vi "Array(DBL)ToFile_v2.vi"(0 "name_base":string="seqOUT", 1 "identifier(\"\")":string="trial01~000", 3 "extension (\".psv\")":string=".psv", 4 "1D-Array":dbl[](array[numeric])=[25.0, 55.0, 73.0, 90.0, 25.0, 55.0, 73.0, 90.0, 25.0, 55.0, 73.0, 90.0, 25.0, 55.0, 73.0, 90.0, 25.0, 55.0, 73.0, 90.0, 25.0, 55.0, 73.0, 90.0, 25.0, 55.0, 73.0, 90.0, 25.0, 55.0, 73.0, 90.0, 25.0, 55.0, 73.0, 90.0, 25.0, 55.0, 73.0, 90.0, 25.0, 55.0, 73.0, 90.0, 25.0, 55.0, 73.0, 90.0, 25.0, 55.0, 73.0, 90.0, 25.0, 55.0, 73.0, 90.0, 25.0, 55.0, 73.0, 90.0, 25.0, 55.0, 73.0, 90.0, 25.0, 55.0, 73.0, 90.0, 25.0, 55.0, 73.0, 90.0, 25.0, 55.0, 73.0, 90.0, 25.0, 55.0, 73.0, 90.0, 25.0, 55.0, 73.0, 90.0, 25.0, 55.0, 73.0, 90.0, 25.0, 55.0, 73.0, 90.0, 25.0, 55.0, 73.0, 90.0, 25.0, 55.0, 73.0, 90.0, 25.0, 55.0, 73.0, 90.0, 25.0, 55.0, 73.0, 90.0, 25.0, 55.0, 73.0, 90.0, 25.0, 55.0, 73.0, 90.0, 25.0, 55.0, 73.0, 90.0, 25.0, 55.0, 73.0, 90.0, 25.0, 55.0, 73.0, 90.0, 25.0, 55.0, 73.0, 90.0, 25.0, 55.0, 73.0, 90.0, 25.0, 55.0, 73.0, 90.0, 25.0, 55.0, 73.0, 90.0, 25.0, 55.0, 73.0, 90.0, 25.0, 55.0, 73.0, 90.0, 25.0, 55.0, 73.0, 90.0, 25.0, 55.0, 73.0, 90.0, 25.0, 55.0, 73.0, 90.0, 25.0, 55.0, 73.0, 90.0, 25.0, 55.0, 73.0, 90.0, 25.0, 55.0, 73.0, 90.0, 25.0, 55.0, 73.0, 90.0, 25.0, 55.0, 73.0, 90.0, 25.0, 55.0, 73.0, 90.0, 25.0, 55.0, 73.0, 90.0, 25.0, 55.0, 73.0, 90.0, 25.0, 55.0, 73.0, 90.0, 25.0, 55.0, 73.0, 90.0, 25.0, 55.0, 73.0, 90.0, 25.0, 55.0, 73.0, 90.0, 25.0, 55.0, 73.0, 90.0, 25.0, 55.0, 73.0, 90.0, 25.0, 55.0, 73.0, 90.0, 25.0, 55.0, 73.0, 90.0, 25.0, 55.0, 73.0, 90.0, 25.0, 55.0, 73.0, 90.0, 25.0, 55.0, 73.0, 90.0, 25.0, 55.0, 73.0, 90.0, 25.0, 55.0, 73.0, 90.0, 25.0, 55.0, 73.0, 90.0, 25.0, 55.0, 73.0, 90.0, 25.0, 55.0, 73.0, 90.0, 25.0, 55.0, 73.0, 90.0, 25.0, 55.0, 73.0, 90.0, 25.0, 55.0, 73.0, 90.0, 25.0, 55.0, 73.0, 90.0, 25.0, 55.0, 73.0, 90.0, 25.0, 55.0, 73.0, 90.0, 25.0, 55.0, 73.0, 90.0, 25.0, 55.0, 73.0, 90.0, 25.0, 55.0, 73.0, 90.0, 25.0, 55.0, 73.0, 90.0, 25.0, 55.0, 73.0, 90.0, 25.0, 55.0, 73.0, 90.0, 25.0, 55.0, 73.0, 90.0, 25.0, 55.0, 73.0, 90.0, 25.0, 55.0, 73.0, 90.0, 25.0, 55.0, 73.0, 90.0, 25.0, 55.0, 73.0, 90.0, 25.0, 55.0, 73.0, 90.0, 25.0, 55.0, 73.0, 90.0, 25.0, 55.0, 73.0, 90.0, 25.0, 55.0, 73.0, 90.0, 25.0, 55.0, 73.0, 90.0, 25.0, 55.0, 73.0, 90.0, 25.0, 55.0, 73.0, 90.0, 25.0, 55.0, 73.0, 90.0, 25.0, 55.0, 73.0, 90.0, 25.0, 55.0, 73.0, 90.0, 25.0, 55.0, 73.0, 90.0, 25.0, 55.0, 73.0, 90.0, 25.0, 55.0, 73.0, 90.0, 25.0, 55.0, 73.0, 90.0, 25.0, 55.0, 73.0, 90.0, 25.0, 55.0, 73.0, 90.0, 25.0, 55.0, 73.0, 90.0, 25.0, 55.0, 73.0, 90.0, 25.0, 55.0, 73.0, 90.0, 25.0, 55.0, 73.0, 90.0, 25.0, 55.0, 73.0, 90.0, 25.0, 55.0, 73.0, 90.0, 25.0, 55.0, 73.0, 90.0, 25.0, 55.0, 73.0, 90.0, 25.0, 55.0, 73.0, 90.0, 25.0, 55.0, 73.0, 90.0, 25.0, 55.0, 73.0, 90.0, 25.0, 55.0, 73.0, 90.0, 25.0, 55.0, 73.0, 90.0, 25.0, 55.0, 73.0, 90.0, 25.0, 55.0, 73.0, 90.0, 25.0, 55.0, 73.0, 90.0, 25.0, 55.0, 73.0, 90.0, 25.0, 55.0, 73.0, 90.0, 25.0, 55.0, 73.0, 90.0, 25.0, 55.0, 73.0, 90.0, 25.0, 55.0, 73.0, 90.0, 25.0, 55.0, 73.0, 90.0, 25.0, 55.0, 73.0, 90.0, 25.0, 55.0, 73.0, 90.0, 25.0, 55.0, 73.0, 90.0, 25.0, 55.0, 73.0, 90.0, 25.0, 55.0, 73.0, 90.0, 25.0, 55.0, 73.0, 90.0, 25.0, 55.0, 73.0, 90.0, 25.0, 55.0, 73.0, 90.0, 25.0, 55.0, 73.0, 90.0, 25.0, 55.0, 73.0, 90.0, 25.0, 55.0, 73.0, 90.0, 25.0, 55.0, 73.0, 90.0, 25.0, 55.0, 73.0, 90.0, 25.0, 55.0, 73.0, 90.0, 25.0, 55.0, 73.0, 90.0, 25.0, 55.0, 73.0, 90.0, 25.0, 55.0, 73.0, 90.0, 25.0, 55.0, 73.0, 90.0, 25.0, 55.0, 73.0, 90.0, 25.0, 55.0, 73.0, 90.0, 25.0, 55.0, 73.0, 90.0, 25.0, 55.0, 73.0, 90.0, 25.0, 55.0, 73.0, 90.0, 25.0, 55.0, 73.0, 90.0, 25.0, 55.0, 73.0, 90.0, 25.0, 55.0, 73.0, 90.0, 25.0, 55.0, 73.0, 90.0, 25.0, 55.0, 73.0, 90.0, 25.0, 55.0, 73.0, 90.0, 25.0, 55.0, 73.0, 90.0, 25.0, 55.0, 73.0, 90.0, 25.0, 55.0, 73.0, 90.0, 25.0, 55.0, 73.0, 90.0, 25.0, 55.0, 73.0, 90.0, 25.0, 55.0, 73.0, 90.0, 25.0, 55.0, 73.0, 90.0, 25.0, 55.0, 73.0, 90.0, 25.0, 55.0, 73.0, 90.0, 25.0, 55.0, 73.0, 90.0, 25.0, 55.0, 73.0, 90.0, 25.0, 55.0, 73.0, 90.0, 25.0, 55.0, 73.0, 90.0, 25.0, 55.0, 73.0, 90.0, 25.0, 55.0, 73.0, 90.0, 25.0, 55.0, 73.0, 90.0, 25.0, 55.0, 73.0, 90.0, 25.0, 55.0, 73.0, 90.0, 25.0, 55.0, 73.0, 90.0, 25.0, 55.0, 73.0, 90.0, 25.0, 55.0, 73.0, 90.0, 25.0, 55.0, 73.0, 90.0, 25.0, 55.0, 73.0, 90.0, 25.0, 55.0, 73.0, 90.0, 25.0, 55.0, 73.0, 90.0, 25.0, 55.0, 73.0, 90.0, 25.0, 55.0, 73.0, 90.0, 25.0, 55.0, 73.0, 90.0, 25.0, 55.0, 73.0, 90.0, 25.0, 55.0, 73.0, 90.0, 25.0, 55.0, 73.0, 90.0, 25.0, 55.0, 73.0, 90.0, 25.0, 55.0, 73.0, 90.0, 25.0, 55.0, 73.0, 90.0, 25.0, 55.0, 73.0, 90.0, 25.0, 55.0, 73.0, 90.0, 25.0, 55.0, 73.0, 90.0, 25.0, 55.0, 73.0, 90.0, 25.0, 55.0, 73.0, 90.0, 25.0, 55.0, 73.0, 90.0, 25.0, 55.0, 73.0, 90.0, 25.0, 55.0, 73.0, 90.0, 25.0, 55.0, 73.0, 90.0, 25.0, 55.0, 73.0, 90.0, 25.0, 55.0, 73.0, 90.0, 25.0, 55.0, 73.0, 90.0, 25.0, 55.0, 73.0, 90.0, 25.0, 55.0, 73.0, 90.0, 25.0, 55.0, 73.0, 90.0, 25.0, 55.0, 73.0, 90.0, 25.0, 55.0, 73.0, 90.0, 25.0, 55.0, 73.0, 90.0, 25.0, 55.0, 73.0, 90.0, 25.0, 55.0, 73.0, 90.0, 25.0, 55.0, 73.0, 90.0, 25.0, 55.0, 73.0, 90.0, 25.0, 55.0, 73.0, 90.0, 25.0, 55.0, 73.0, 90.0, 25.0, 55.0, 73.0, 90.0, 25.0, 55.0, 73.0, 90.0, 25.0, 55.0, 73.0, 90.0, 25.0, 55.0, 73.0, 90.0, 25.0, 55.0, 73.0, 90.0, 25.0, 55.0, 73.0, 90.0, 25.0, 55.0, 73.0, 90.0, 25.0, 55.0, 73.0, 90.0, 25.0, 55.0, 73.0, 90.0, 25.0, 55.0, 73.0, 90.0, 25.0, 55.0, 73.0, 90.0, 25.0, 55.0, 73.0, 90.0, 25.0, 55.0, 73.0, 90.0, 25.0, 55.0, 73.0, 90.0, 25.0, 55.0, 73.0, 90.0, 25.0, 55.0, 73.0, 90.0, 25.0, 55.0, 73.0, 90.0, 25.0, 55.0, 73.0, 90.0, 25.0, 55.0, 73.0, 90.0, 25.0, 55.0, 73.0, 90.0, 25.0, 55.0, 73.0, 90.0, 25.0, 55.0, 73.0, 90.0, 25.0, 55.0, 73.0, 90.0, 25.0, 55.0, 73.0, 90.0, 25.0, 55.0, 73.0, 90.0, 25.0, 55.0, 73.0, 90.0, 25.0, 55.0, 73.0, 90.0, 25.0, 55.0, 73.0, 90.0, 25.0, 55.0, 73.0, 90.0, 25.0, 55.0, 73.0, 90.0, 25.0, 55.0, 73.0, 90.0, 25.0, 55.0, 73.0, 90.0, 25.0, 55.0, 73.0, 90.0, 25.0, 55.0, 73.0, 90.0, 25.0, 55.0, 73.0, 90.0, 25.0, 55.0, 73.0, 90.0, 25.0, 55.0, 73.0, 90.0, 25.0, 55.0, 73.0, 90.0, 25.0, 55.0, 73.0, 90.0, 25.0, 55.0, 73.0, 90.0, 25.0, 55.0, 73.0, 90.0, 25.0, 55.0, 73.0, 90.0, 25.0, 55.0, 73.0, 90.0] format="%_8f", 5 "2D-Array":dbl[][](array[numeric])=array100x100[10000 elements] format="%_8f", 7 "Array Type (2D)":enum16{"2D", "row", "column"}(ring), 8 "Child Directory":path=path "SEQUENCES/OUT", 9 "delimiter (\"|\")":string="|", 11 "data format (DBL)":string="%.8f", 12 "Parent Directory":path=path "C:/misc/LabVIEW/FILES", 13 "Filename Collision Handling":T1(ring)) -> (20 "target_filepath":path=path "C:/misc/LabVIEW/FILES/SEQUENCES/OUT/seqOUT_trial01.psv", 23 "Saved":bool=TRUE, 25 "data_string":string="25\r\n55\r\n73\r\n90\r\n25\r\n55\r\n73\r\n90\r\n25\r\n55\r\n73\r\n90\r\n25\r\n55\r\n73\r\n90\r\n25\r\n55\r\n73\r\n90\r\n25\r\n55\r\n73\r\n90\r\n25\r\n55\r\n73\r\n90\r\n25\r\n55\r\n73\r\n90\r\n25\r\n55\r\n73\r\n90\r\n25\r\n55\r\n73\r\n90\r\n25\r\n55\r\n73\r\n90\r\n25\r\n55\r\n73\r\n90\r\n25\r\n55\r\n73\r\n90\r\n25\r\n55\r\n73\r\n90\r\n25\r\n55\r\n73\r\n90\r\n25\r\n55\r\n73\r\n90\r\n25\r\n55\r\n73\r\n90\r\n25\r\n55\r\n73\r\n90\r\n25\r\n55\r\n73\r\n90\r\n25\r\n55\r\n73\r\n90\r\n25\r\n55\r\n73\r\n90\r\n25\r\n55\r\n73\r\n90\r\n25\r\n55\r\n73\r\n90\r\n25\r\n55\r\n73\r\n90\r\n25\r\n55\r\n73\r\n90\r\n25\r\n55\r\n73\r\n90\r\n25\r\n55\r\n73\r\n90\r\n25\r\n55\r\n73\r\n90\r\n25\r\n55\r\n73\r\n90\r\n25\r\n55\r\n73\r\n90\r\n25\r\n55\r\n73\r\n90\r\n25\r\n55\r\n73\r\n90\r\n25\r\n55\r\n73\r\n90\r\n25\r\n55\r\n73\r\n90\r\n25\r\n55\r\n73\r\n90\r\n25\r\n55\r\n73\r\n90\r\n25\r\n55\r\n73\r\n90\r\n25\r\n55\r\n...")   [LabVIEW 2014]
panel:
  in  "?":enum32{"MAIN", "DATA"}(tab)
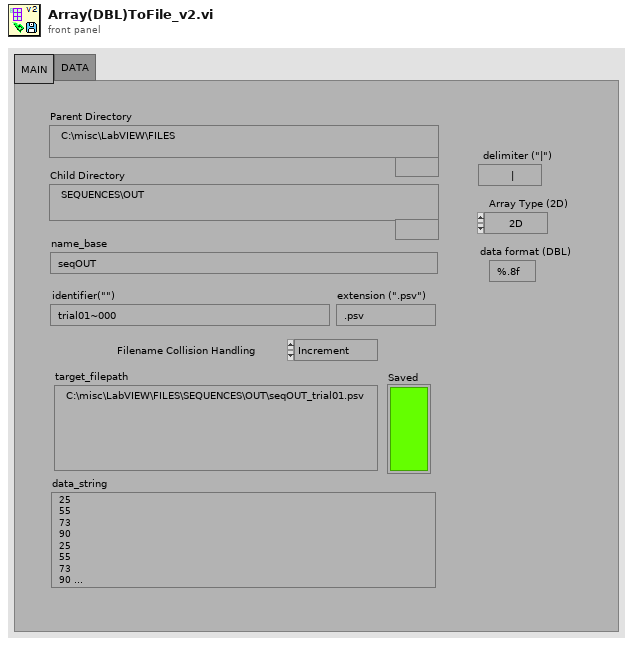
[diagram p1: front panel]
types:
  T1 = enum16{"Increment", "Overwrite", "Treat as Error"}
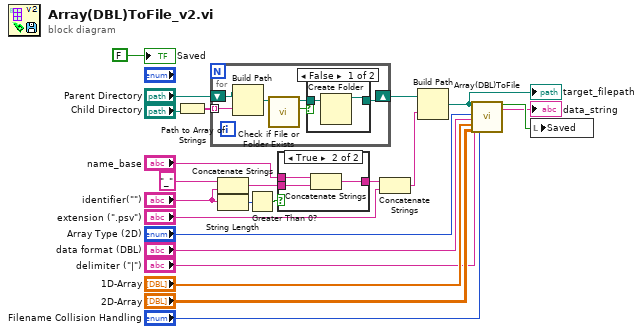
[diagram p0: block diagram]
diagram:
  n1 = Path to Array of Strings(0:"Child Directory") -> (2:w21:string[])  [unwired: 1 out]
  n2 = for {
    tunnel: w21 -> [w28] mode=indexing
    shift-right: [w24] -> w19
    shift-left: "Parent Directory" -> [w29]
    n3 = Build Path(base path=w29, name or relative path=w28) -> (appended path=w27:path)
    n4 = call <vilib>:"Check if File or Folder Exists.vi"("path"=w27) -> ("file or folder exists?"=w26:bool, "dup path"=w25:path)  [unwired: 8 in, 1 out]
    n5 = case shown="False" w26 {
      tunnel: w25 -> [w31 w32]
      tunnel: [w30 w32] -> w24
      frame False {
        n6 = Create Folder(path (use dialog)=w31) -> (created path=w30:path)  [unwired: 2 in, 2 out]
      }
      frame True {
      }
    }
  }
  n7 = Concatenate Strings("_" ("name_delimiter (\"_\")"), "identifier(\"\")") -> (w11:string)
  n8 = String Length(string="identifier(\"\")") -> (length=w15:i32)
  n9 = Greater Than 0?(x=w15) -> (x > 0?=w14:bool)
  n10 = case shown="True" w14 {
    tunnel: w11 -> [_ w35]
    tunnel: "name_base" -> [w33 w36]
    tunnel: [w33 w34] -> w9
    frame False {
    }
    frame True {
      n11 = Concatenate Strings(w36, w35) -> (w34:string)
    }
  }
  n12 = Concatenate Strings(w9, "extension (\".psv\")") -> (w7:string)
  n13 = Build Path(base path=w19, name or relative path=w7) -> (appended path=w18:path)
  "target_filepath" <- w18
  n14 = call "Array(DBL)ToFile.vi"("path"=w18, "Array Type (2D)"="Array Type (2D)", "data format (DBL)"="data format (DBL)", "Array(1D)"="1D-Array", "Array(2D)"="2D-Array", "delimiter (\"|\")"="delimiter (\"|\")", "Filename Collision Handling"="Filename Collision Handling") -> ("Saved"=w17:bool, "File content"=→"data_string":string)  [unwired: 11 in]
  n15 = local write "Saved"(w17) -> ()
  "Saved" <- FALSE
